vi "Read Temperature results.vi"(8 "error in (no error)":errorcluster, 11 "IV in":refnum<class "IV.lvclass">) -> (0 "error out":errorcluster, 2 "Temperature results":refnum<class "Acquired Result.lvclass">[](array[class]), 3 "IV out":refnum<class "IV.lvclass">)   [LabVIEW 2021, in "IV.lvclass"]
uses:
  IV.lvclass
  Libraries/Instruments/Results/Acquired Result/Acquired Result.lvclass
  IV.lvclass/IV.ctl
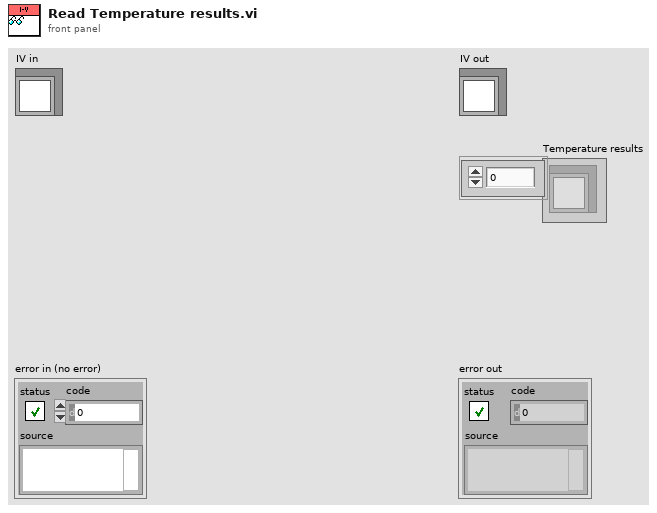
[diagram p1: front panel]
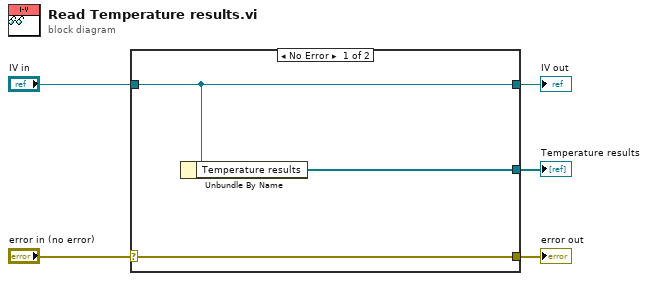
[diagram p0: block diagram]
diagram:
  n1 = case shown="No Error" "error in (no error)" {
    selector: "error in (no error)" -> [w8 w9]
    tunnel: [w8 w9] -> w4
    tunnel: [w7 w10] -> w2
    tunnel: "IV in" -> [w7 w10]
    tunnel: [w6 _] -> w1
    frame No Error {
      n2 = Unbundle By Name(w7) -> ("Temperature results"=w6:refnum<class "Acquired Result.lvclass">[])
    }
    frame Error {
    }
  }
  "error out" <- w4
  "IV out" <- w2
  "Temperature results" <- w1
